vi "File.Find Subdir using pattern.vi"(8 "error in (no error)":errorcluster, 10 "Pattern":string, 11 "Folder":path) -> (0 "error out":errorcluster, 3 "Found Folders":path[](array[path]))   [LabVIEW 2019]
uses:
  <vilib>/KATE/Files/File Utils.lvlib
panel:
  out "Found":bool
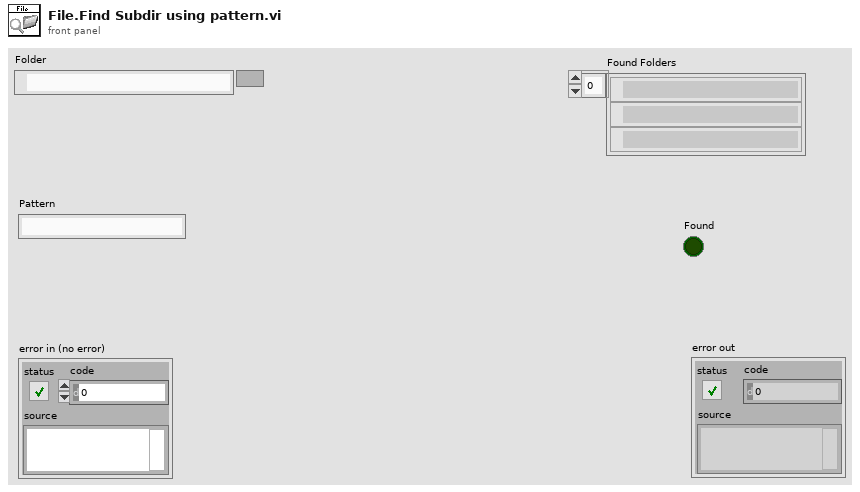
[diagram p1: front panel]
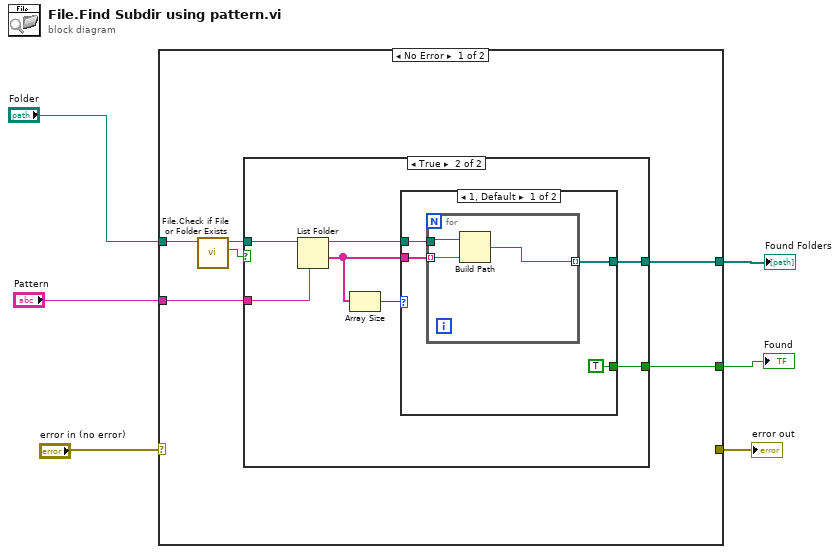
[diagram p0: block diagram]
diagram:
  n1 = case shown="No Error" "error in (no error)" {
    selector: "error in (no error)" -> [_ w27]
    tunnel: "Folder" -> [w10 _]
    tunnel: [w12 _] -> w5
    tunnel: "Pattern" -> [w11 _]
    tunnel: [_ w27] -> w2
    tunnel: [w7 _] -> w1
    frame No Error {
      n2 = call <vilib>:"File.Check if File or Folder Exists.vi"("Path"=w10) -> ("Exists"=w8:bool, "Dup Path"=w9:path)  [unwired: 6 in, 3 out]
      n3 = case shown="True" w8 {
        tunnel: [_ w18] -> w12
        tunnel: w11 -> [_ w15]
        tunnel: w9 -> [_ w17]
        tunnel: [_ w13] -> w7
        frame False {
        }
        frame True {
          n4 = List Folder(path=w17, pattern=w15) -> (path out=w19:path, folder names=w14:string[])  [unwired: 2 in, 2 out]
          n5 = Array Size(array=w14) -> (size(s)=w16:i32)
          n6 = case shown="1, Default" w16 {
            tunnel: w19 -> [w23 _]
            tunnel: [w20 _] -> w18
            tunnel: w14 -> [w22 _]
            tunnel: [TRUE _] -> w13
            frame 1, Default {
              n7 = for {
                tunnel: w23 -> [w25]
                tunnel: w22 -> [w26] mode=indexing
                tunnel: [w24] -> w20 mode=indexing
                n8 = Build Path(base path=w25, name or relative path=w26) -> (appended path=w24:path)
              }
            }
            frame 0 {
            }
          }
        }
      }
    }
    frame Error {
    }
  }
  "Found Folders" <- w5
  "error out" <- w2
  "Found" <- w1
